vi "UDP_Search.vi"() -> (2 "Connect?":bool, 3 "Connection ID Out":T1)   [LabVIEW 2017, in "GL860_Driver.lvlib"]
uses:
  GL860_Driver.lvlib
  Driver/ConnectionID.ctl
  Sub/UDP_Packet.ctl
  Driver/GLdrv_Open_TCPIP.vi
panel:
  out "Msg":u16(ring) items=["機器検索中..."]
  in  "FirstCall":bool
  in  "ポート":u16=8023
  in  "検索":bool
  in  "キャンセル":bool
  in  "connect":bool
  in  "List":i32(listbox)
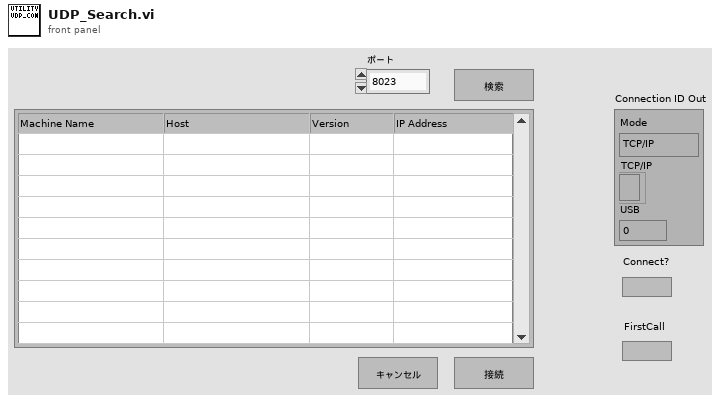
[diagram p1: front panel]
types:
  T1 = typedef "ConnectionID.ctl" = cluster{"Mode":enum16{"TCP/IP", "USB"}, "TCP/IP":refnum<k5>, "USB":i32}
  T2 = typedef "UDP_Packet.ctl" = cluster{"Name":string, "ID":u32, "BC":bool, "Res":bool, "Command":u32, "Param":string}
  T3 = cluster{"Machine":string, "Firm":string, "Host":string, "IP":string, "Count":u32, "IP_Busy":u32, "USB":u32, "AnalogCH":u32, "AmpUnit":u32, "Sens":string, "Name":string}[]
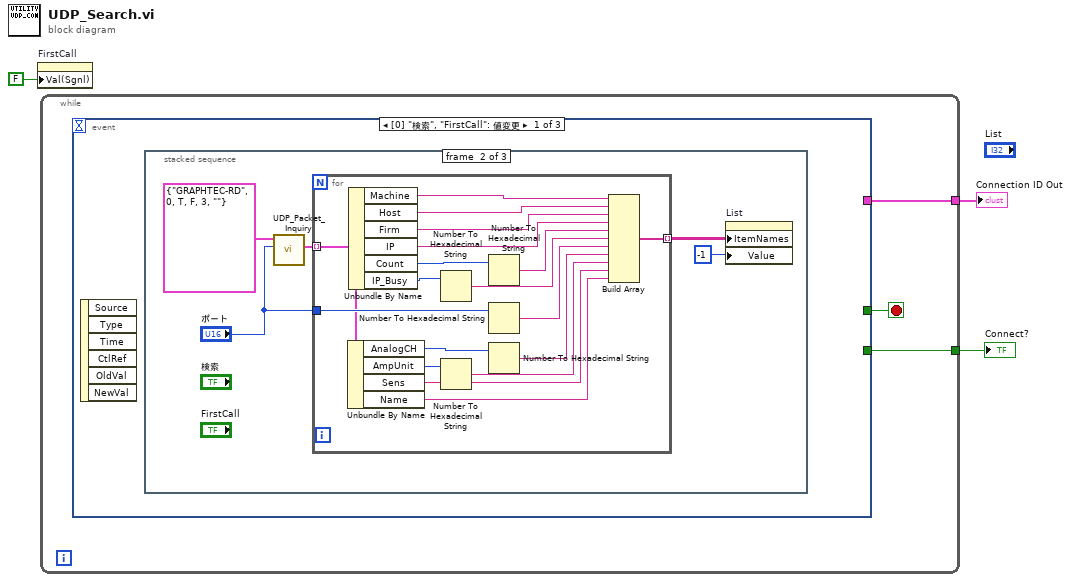
[diagram p0: block diagram]
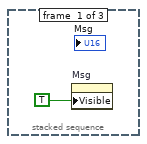
[diagram p2: hidden frame]
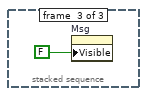
[diagram p3: hidden frame]
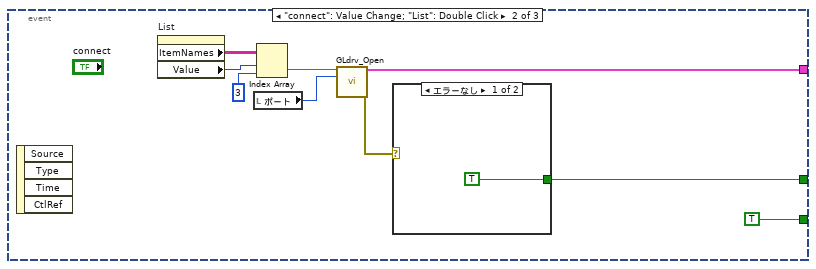
[diagram p4: hidden frame]
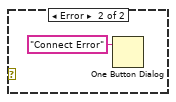
[diagram p5: hidden frame]
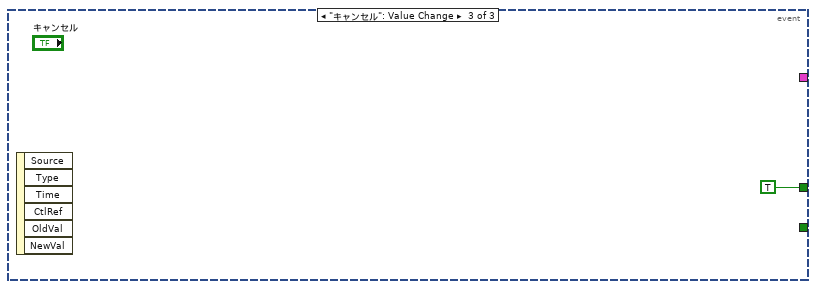
[diagram p6: hidden frame]
diagram:
  n1 = property on="FirstCall" class="Bool （指定）"("Val(Sgnl)"=FALSE ("Value (Signaling)")) -> ()  [unwired: 2 in, 2 out]
  n2 = while {
    tunnel: [w5] -> w3
    tunnel: [w4] -> w2
    stop <- w6 stop-if-true
    n3 = event shown="[0] \"検索\", \"FirstCall\": 値変更" {
      selector: _ -> [_ _ _]
      dyn-events: _ -> [_ _ _]
      timeout: _ -> [_ _ _]
      tunnel: [_ w33 TRUE] -> w6
      tunnel: [_ w36 _] -> w5
      tunnel: [_ TRUE _] -> w4
      event "検索", "FirstCall": Value Change {
        n4 = event-data() -> ()  [unwired: 1 in, 6 out]
        n5 = stacked-sequence {
          frame #0 {
            n6 = property on="Msg" class="Ring （指定）"("Visible"=TRUE) -> ()  [unwired: 2 in, 2 out]
          }
          frame #1 {
            n7 = call "UDP_Packet_Inquiry.vi"("Remote Port"="ポート", "UDP_Packet"=T2 {"Name"="GRAPHTEC-RD", "ID"=0, "BC"=TRUE, "Res"=FALSE, "Command"=3, "Param"=""}) -> ("List"=w12:T3)  [unwired: 9 out]
            n8 = for {
              tunnel: w12 -> [w14] mode=indexing
              tunnel: [w13] -> w9 mode=indexing
              tunnel: "ポート" -> [w21]
              n9 = Unbundle By Name(w14) -> ("AnalogCH"=w15:u32, "AmpUnit"=w16:u32, "Sens"=w17:string, "Name"=w18:string)
              n10 = Unbundle By Name(w14) -> ("Machine"=w28:string, "Host"=w20:string, "Firm"=w19:string, "IP"=w27:string, "Count"=w30:u32, "IP_Busy"=w29:u32)
              n11 = Number To Hexadecimal String(2:w29) -> (0:w25:string)  [unwired: 1 in]
              n12 = Number To Hexadecimal String(2:w16) -> (0:w22:string)  [unwired: 1 in]
              n13 = Number To Hexadecimal String(2:w30) -> (0:w26:string)  [unwired: 1 in]
              n14 = Number To Hexadecimal String(2:w21) -> (0:w24:string)  [unwired: 1 in]
              n15 = Number To Hexadecimal String(2:w15) -> (0:w23:string)  [unwired: 1 in]
              n16 = Build Array(w28, w20, w19, w27, w26, w25, w24, w23, w22, w17, w18) -> (w13:string[])
            }
            n17 = property on="List" class="MCListbox （指定）"("ItemNames"=w9, "Value"=-1 ("List")) -> ()  [unwired: 2 in, 2 out]
          }
          frame #2 {
            n18 = property on="Msg" class="Ring （指定）"("Visible"=FALSE) -> ()  [unwired: 2 in, 2 out]
          }
        }
      }
      event "connect": Value Change; "List": Double Click {
        n19 = event-data() -> ()  [unwired: 1 in, 4 out]
        n20 = property on="List" class="MCListbox （指定）"() -> ("ItemNames"=w40:string[][], "Value"=w39:i32)  [unwired: 2 in, 2 out]
        n21 = local read "ポート"() -> (w35:u16)
        n22 = Index Array(array=w40, index (row)=w39, index (col)=3 ("disabled index (col)")) -> (element=w37:string)
        n23 = call-poly "GLdrv_Open.vi"("address"=w37, "remote port"=w35) -> ("Connection ID"=w36:T1, "error out"=w34:errorcluster)  [unwired: 12 in]
        n24 = case shown="エラーなし" w34 {
          tunnel: [TRUE _] -> w33
          frame No Error {
          }
          frame Error {
            n25 = One Button Dialog(message="Connect Error") -> ()  [unwired: 1 in, 1 out]
          }
        }
      }
      event "キャンセル": Value Change {
        n26 = event-data() -> ()  [unwired: 1 in, 6 out]
      }
    }
  }
  "Connection ID Out" <- w3
  "Connect?" <- w2
